vi "BotSpeak_To_String.vi"() -> ()   [LabVIEW 2014]
panel:
  out "format string":string
  in  "spreadsheet string":string
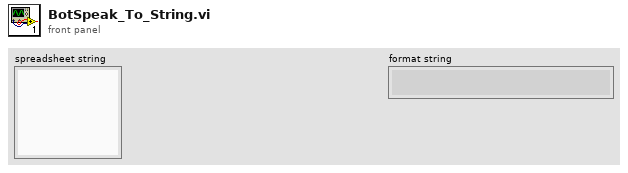
[diagram p1: front panel]
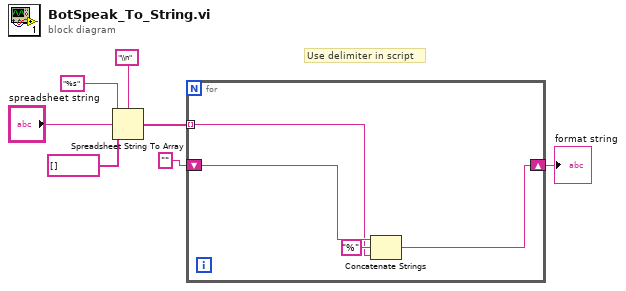
[diagram p0: block diagram]
diagram:
  # "Use delimiter in script"
  n1 = Spreadsheet String To Array(delimiter (Tab)="\\n", format string="%s", spreadsheet string="spreadsheet string", array type (2D Dbl)=string[] []) -> (array=w3:string[])
  n2 = for {
    tunnel: w3 -> [w8] mode=indexing
    shift-right: [w9] -> w1
    shift-left: "" ("format string") -> [w11]
    n3 = Concatenate Strings(w11, "%" ("string"), w8) -> (w9:string)
  }
  "format string" <- w1
